vi "BATTERY EMULATOR.vi"() -> ()   [LabVIEW 2018]
uses:
  17a302df-ff61-441d-8d7b-7ff2f5324251.vi
  <vilib>/xnet/xnet.llb/XNET Create Session (Signal Input Single-point).vi
  <vilib>/xnet/xnet.llb/XNET Read (Signal Single-point).vi
panel:
  in  "READ DATA":bool
  out "CP POWER":string
  out "CP CURRENT":string
  out "CP VOLTAGE":string
  out "CI POWER":string
  out "CI CURRENT":string
  out "CI VOLTAGE":string
  out "CV POWER":string
  out "CV CURRENT":string
  out "CV VOLTAGE":string
  out "CONTROL SELECTION":string
  out "HVHC SELECTION":string
  in  "CP POWER":string
  in  "CP CURRENT":string
  in  "CP VOLTAGE":string
  in  "CI POWER":string
  in  "CI CURRENT":string
  in  "CI VOLTAGE":string
  in  "CV POWER":string
  in  "CV CURRENT":string
  in  "CV VOLTAGE":string
  in  "CONTROL SELECTION":string(combo)
  in  "HVHC SELECTION":string(combo)
  out "Headline":string
  in  "Save Button":bool
  in  "MODEL SELECTION":string(combo)
  # "BATTERY EMULATOR CONTROLS"
  # "BATTERY EMULATOR DATA"
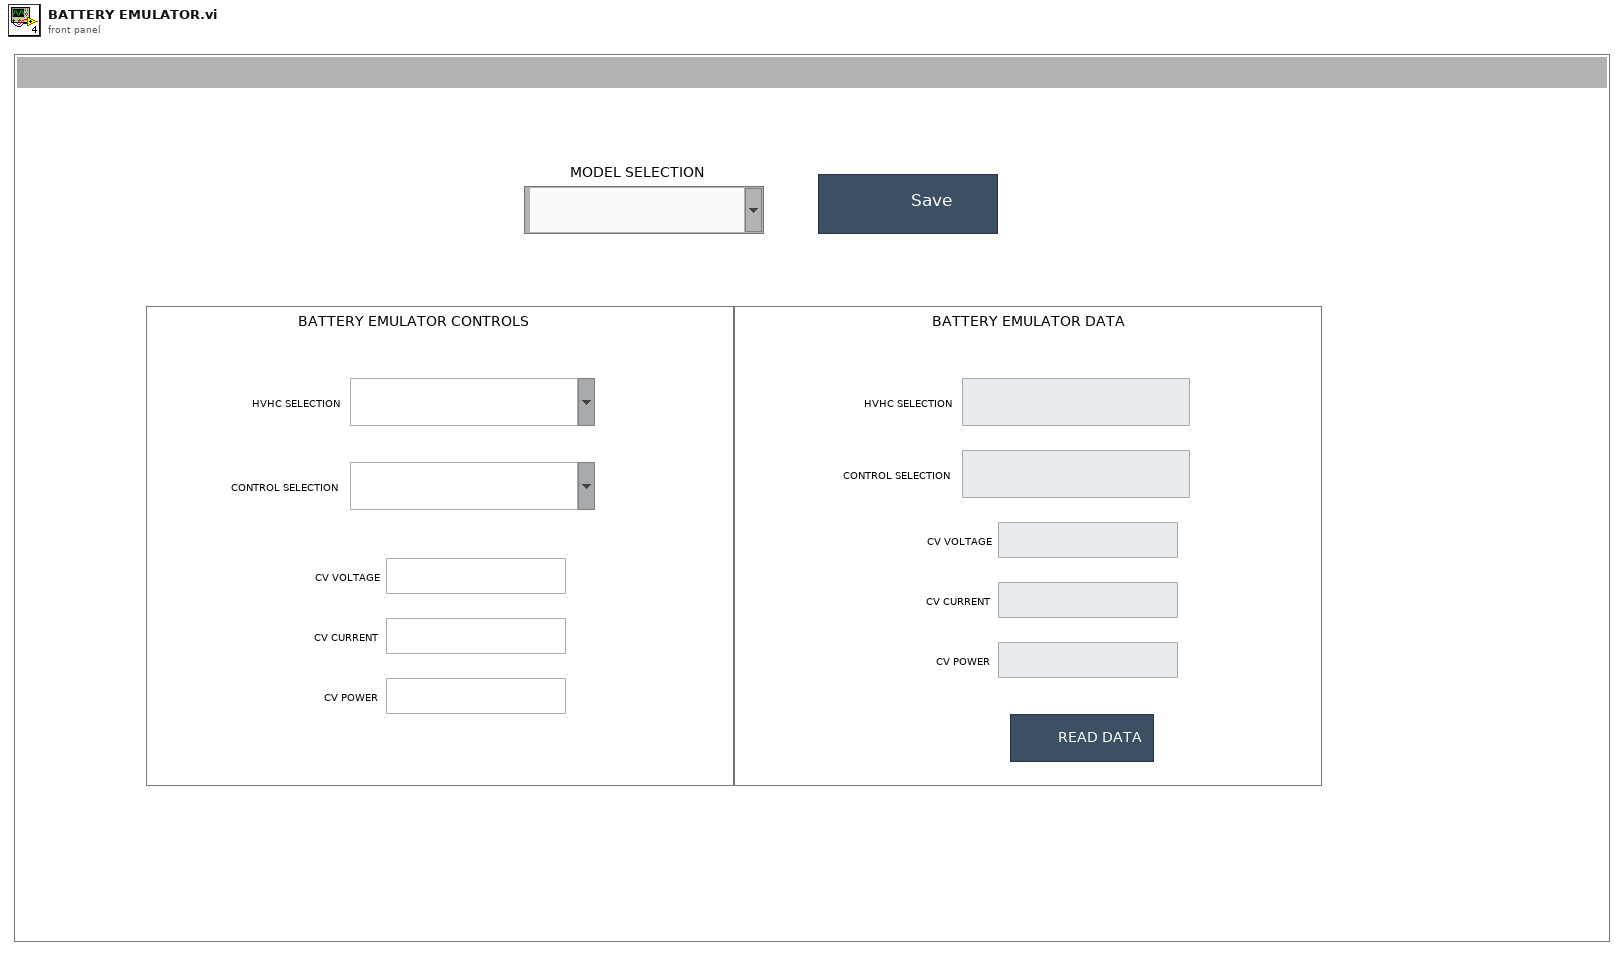
[diagram p1: front panel]
types:
  T1 = enum32{"Invalid", "Standard", "Closed", "Hidden", "Minimized", "Maximized"}
  T2 = enum32{"invalid app kind", "Development System", "Run Time System", "Student Edition", "Embedded LabVIEW", "Evaluation", "Custom"}
  T3 = cluster{"Core":cluster{"Current VI Reference":refnum<vi>, "Close Panel on Exit?":bool}, "Your Boolean data":bool, "Your string data":string, "BATTERY EMULATOR":cluster{"HVHC SELECT":string, "CONTROL SELECTION":string, "CV VOLTAGE":string, "CV CURRENT":string, "CV POWER":string, "CI VOLTAGE":string, "CI CURRENT":string, "CI POWER":string, "CP VOLTAGE":string, "CP CURRENT":string, "CP POWER":string}, "File paths":cluster{"Base file path":path, "Model File path":path}}
  T4 = cluster{"HVHC SELECT":string, "CONTROL SELECTION":string, "CV VOLTAGE":string, "CV CURRENT":string, "CV POWER":string, "CI VOLTAGE":string, "CI CURRENT":string, "CI POWER":string, "CP VOLTAGE":string, "CP CURRENT":string, "CP POWER":string}
  T5 = cluster{"Base file path":path, "Model File path":path}
  T6 = cluster{"Current VI Reference":refnum<vi>, "Close Panel on Exit?":bool}
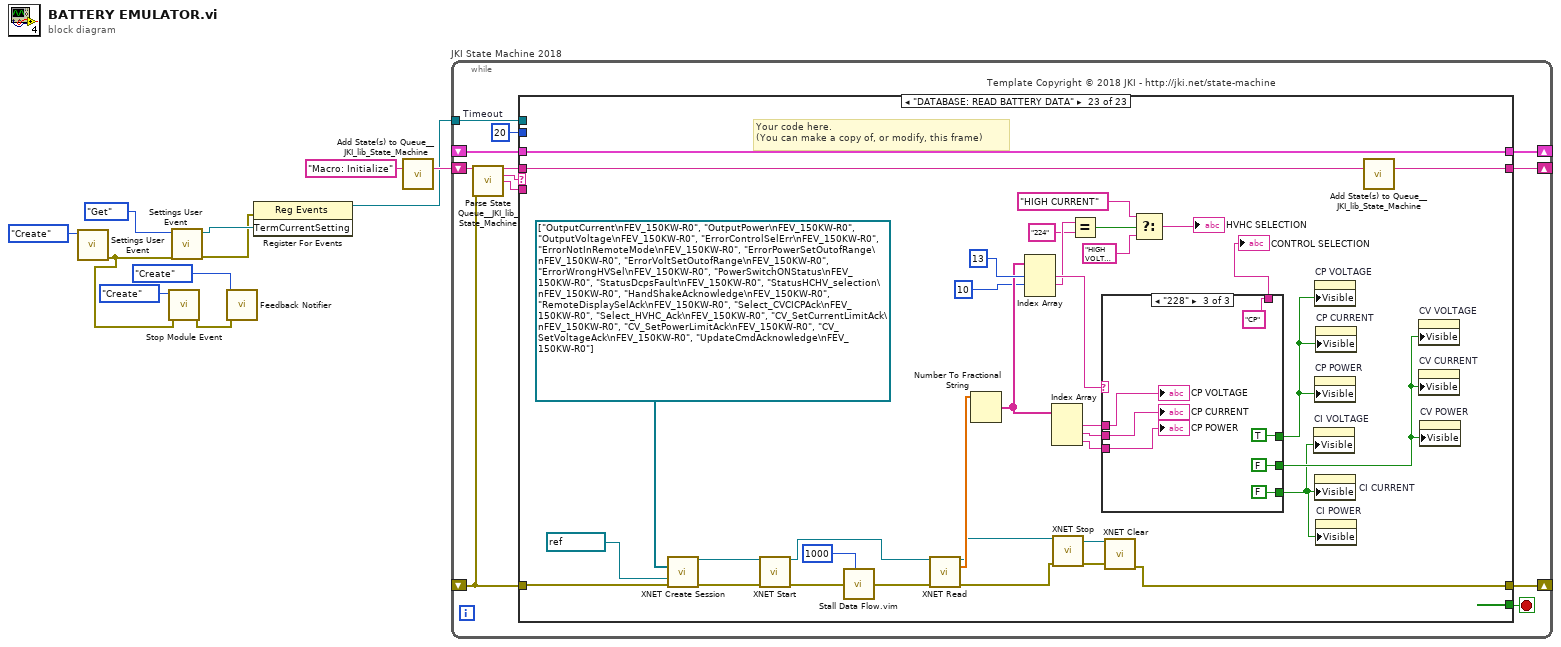
[diagram p0: block diagram]
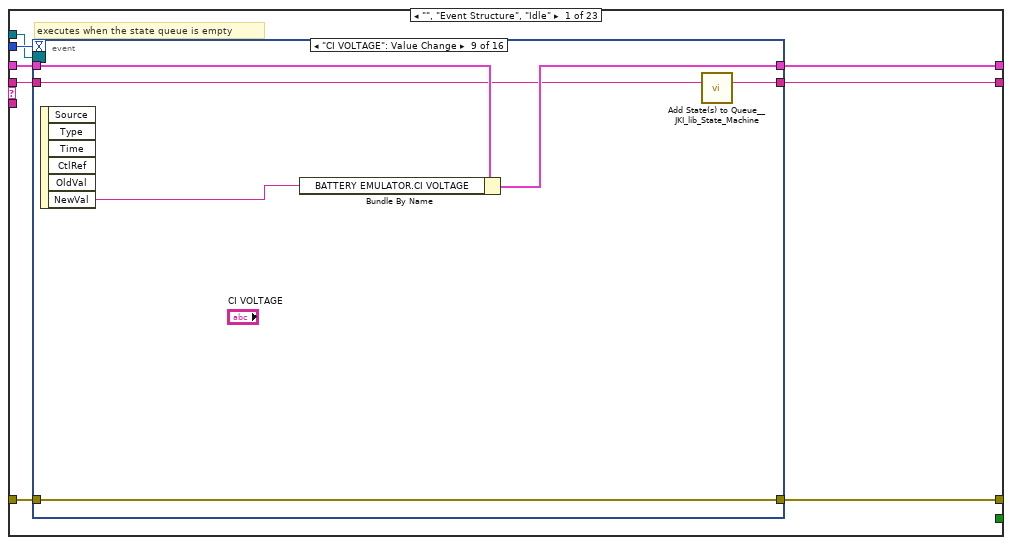
[diagram p2: hidden frame]
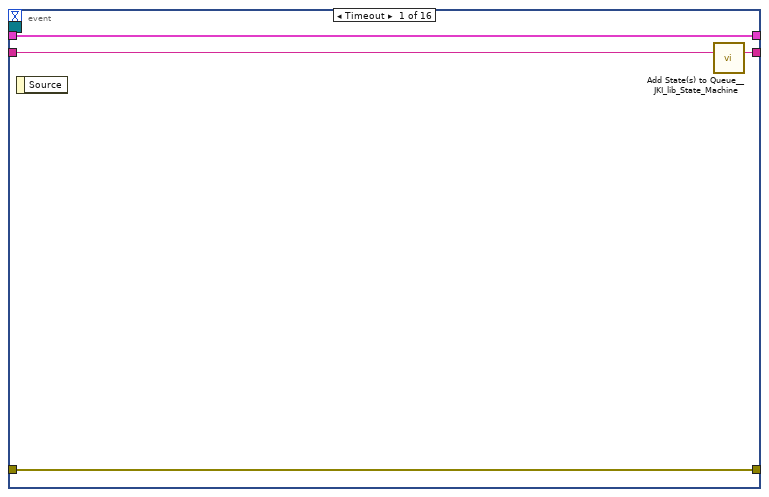
[diagram p3: hidden frame]
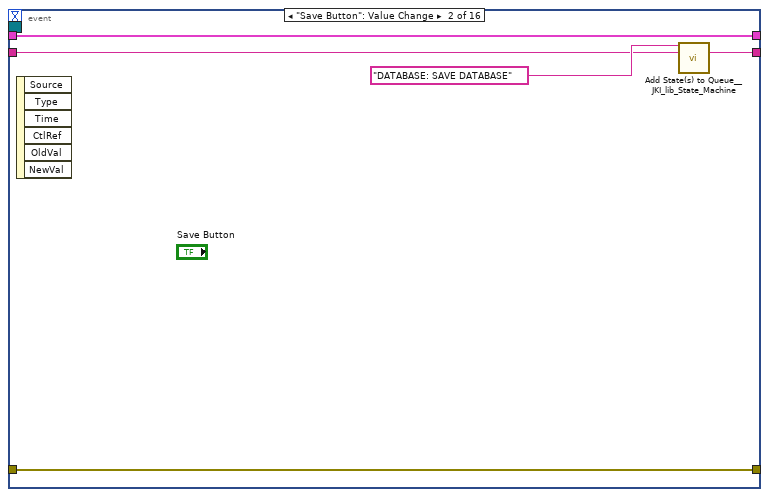
[diagram p4: hidden frame]
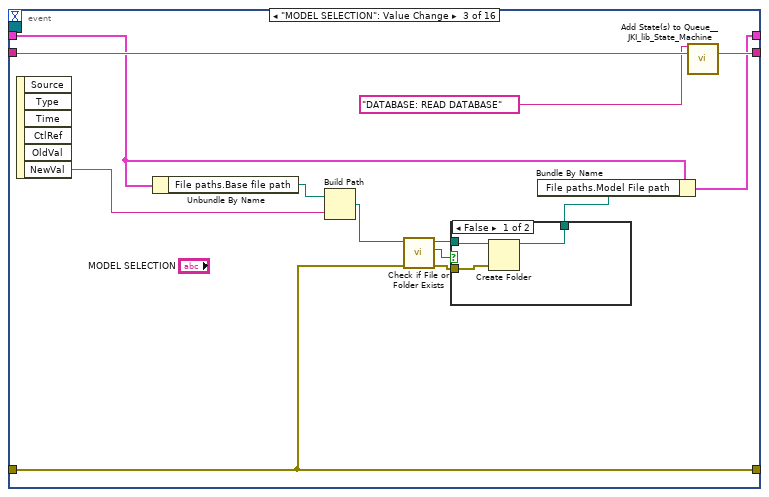
[diagram p5: hidden frame]
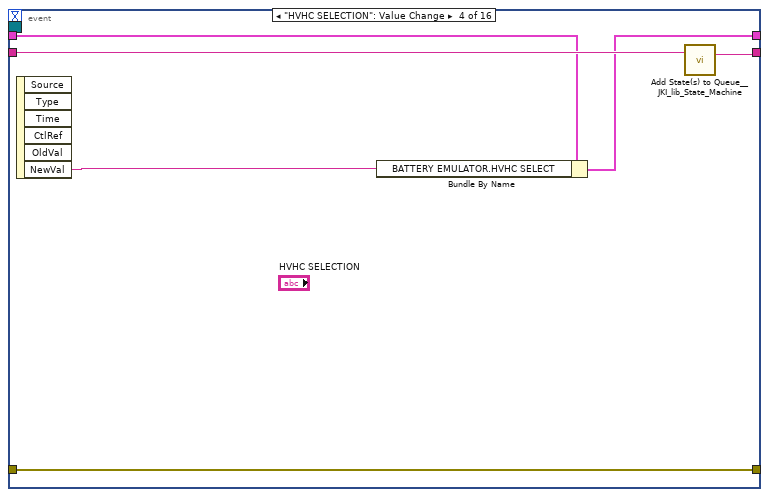
[diagram p7: hidden frame]
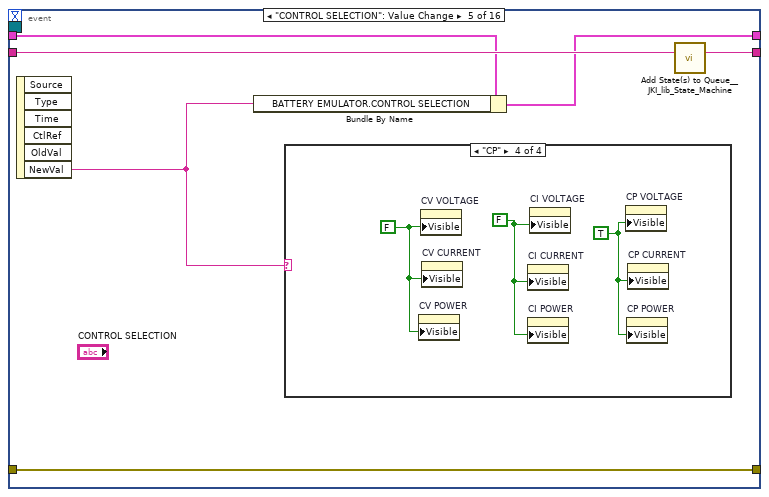
[diagram p8: hidden frame]
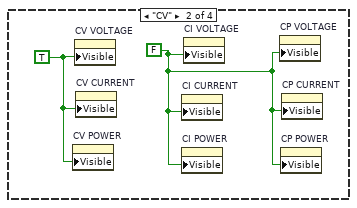
[diagram p10: hidden frame]
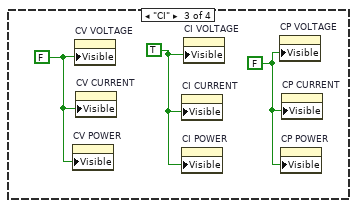
[diagram p11: hidden frame]
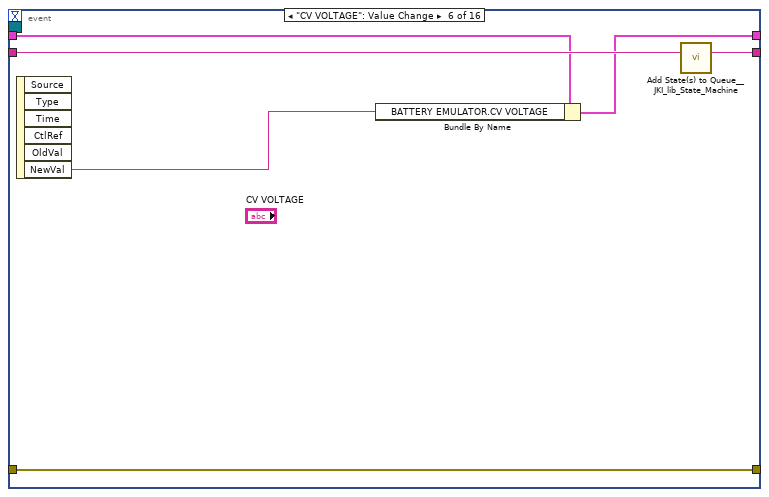
[diagram p12: hidden frame]
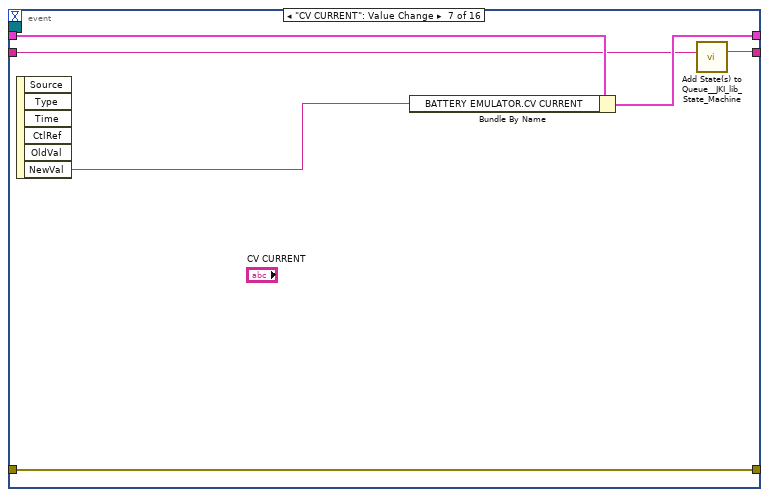
[diagram p13: hidden frame]
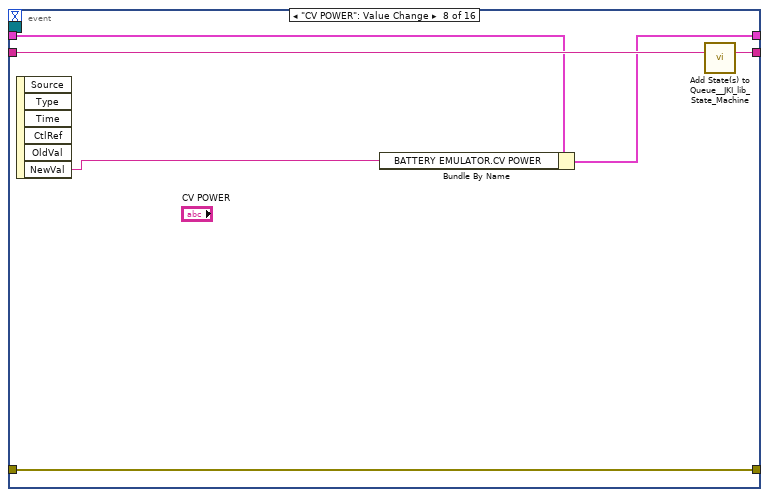
[diagram p14: hidden frame]
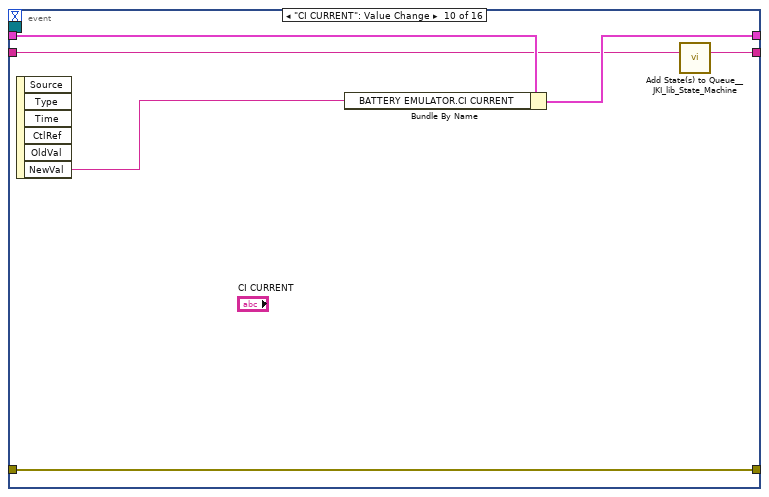
[diagram p15: hidden frame]
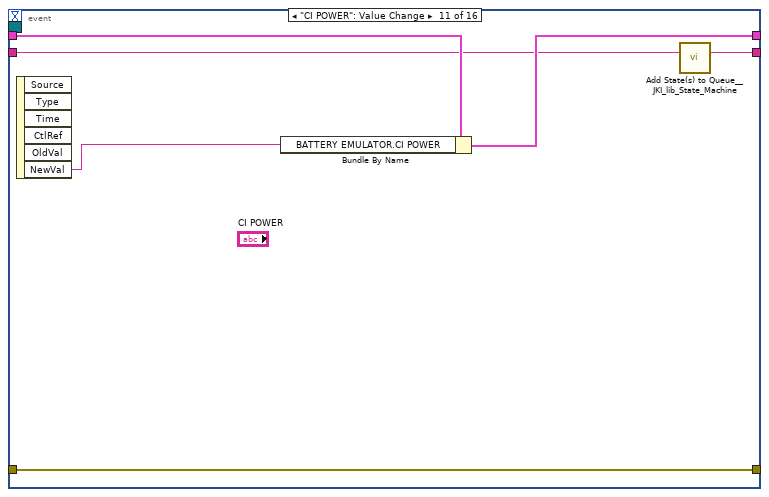
[diagram p16: hidden frame]
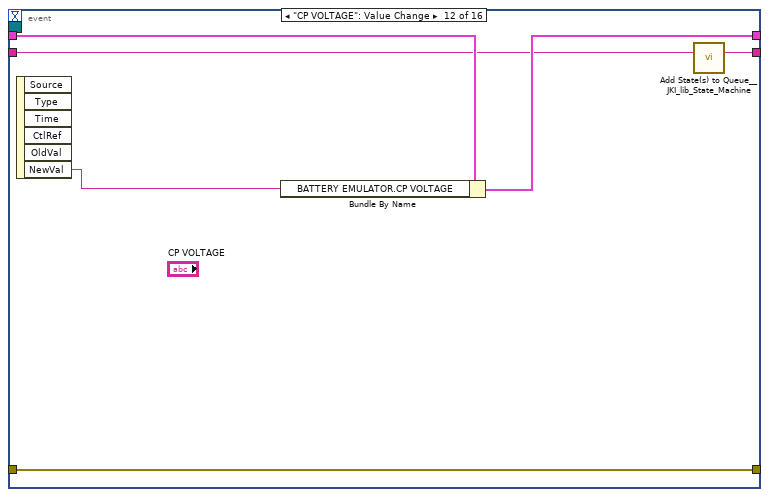
[diagram p17: hidden frame]
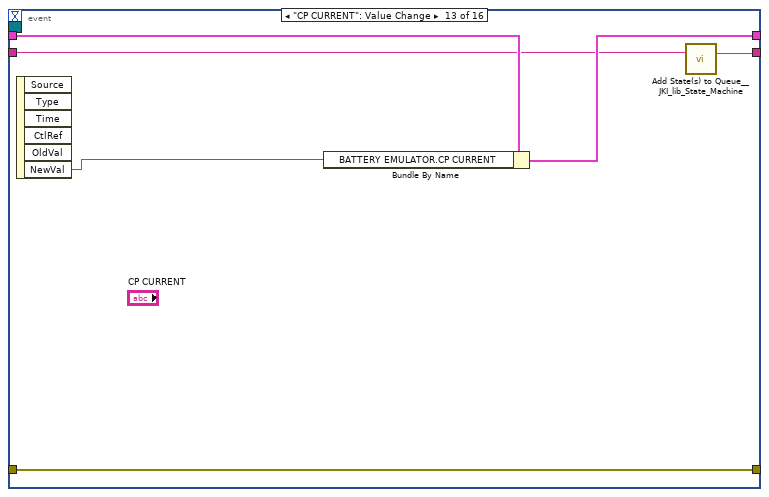
[diagram p18: hidden frame]
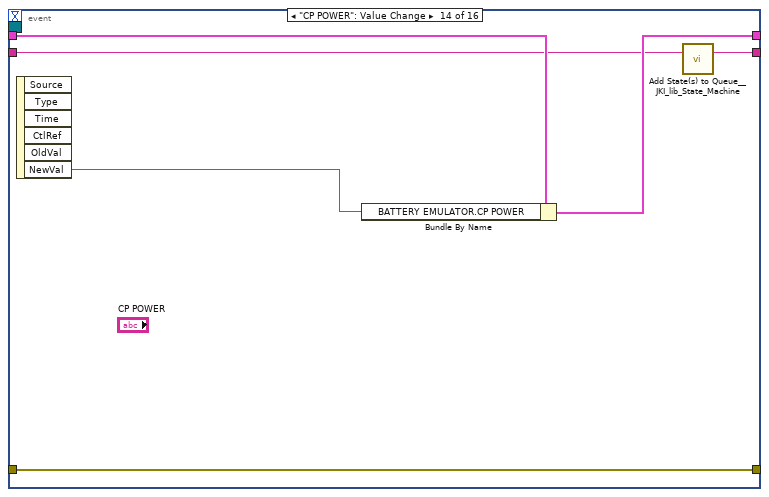
[diagram p19: hidden frame]
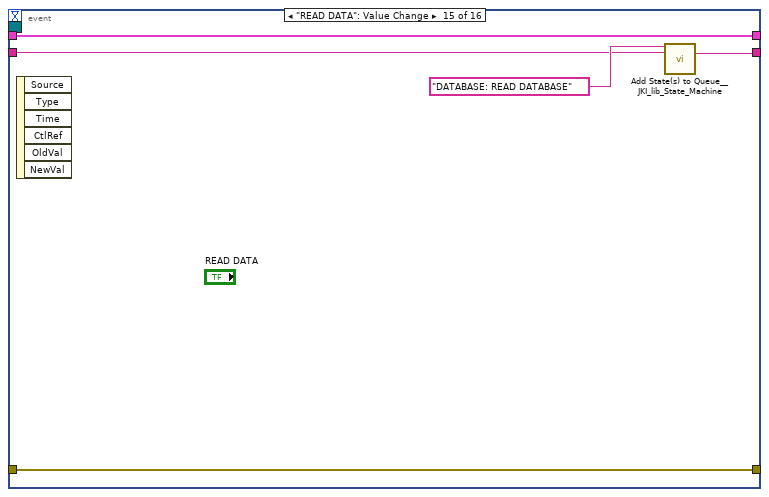
[diagram p20: hidden frame]
diagram:
  n1 = call "Settings User Event.vi"("Action"=enum16{"Create", "Get", "Destroy"}."Create") -> ("error out"=w4:errorcluster)  [unwired: 9 in, 1 out]
  n2 = call "Stop Module Event.vi"("error in (no error)"=w4, "Action"=enum16{"Create", "Get", "Destroy"}."Create") -> ("error out"=w3:errorcluster)  [unwired: 8 in, 1 out]
  n3 = call "Settings User Event.vi"("error in (no error)"=w4, "Action"=enum16{"Create", "Get", "Destroy"}."Get") -> ("error out"=w6:errorcluster, "TermCurrentSetting"=w7:refnum<user-event>)  [unwired: 8 in]
  n4 = call "Feedback Notifier.vi"("error in (no error)"=w3, "Action"=enum16{"Create", "Get", "Destroy"}."Create") -> ()  [unwired: 8 in, 2 out]
  n5 = register-events(error in=w6, w7) -> (reference out=w1:refnum<event-registration>)  [unwired: 1 in, 1 out]
  n6 = call <vilib>:"Add State(s) to Queue__JKI_lib_State_Machine.vi"("State(s) in (\"\")"="Macro: Initialize") -> ("States Out"=w11:string)  [unwired: 14 in]
  n7 = while "JKI State Machine 2018" {
    shift-right: [w16] -> _
    shift-left: _ -> [w15]
    shift-right: [w19] -> _
    shift-left: _ -> [w13]
    shift-right: [w18] -> _
    shift-left: w11 -> [w20]
    tunnel: w1 -> [w12]
    stop <- w17 stop-if-true
    w14 = 20  # Timeout
    # "Template Copyright © 2018 JKI - http://jki.net/state-machine"
    n8 = call <vilib>:"Parse State Queue__JKI_lib_State_Machine.vi"("State Queue"=w20, "Error In (no error)"=w13) -> ("Remaining States"=w22:string, "Current State"=w23:string, "Arguments"=w21:string)  [unwired: 11 in]
    n9 = case shown="\"DATABASE: READ BATTERY DATA\"" w23 {
      selector: w23 -> [_ _ w147 _ _ _ _ _ _ _ _ _ _ _ _ _ _ _ _ _ _ _ _]
      tunnel: w22 -> [w31 w146 w151 w170 w176 w181 w185 w194 w200 w204 w208 w214 w218 w233 w239 w250 w319 w324 w334 w338 w348 w373 w408]
      tunnel: w21 -> [_ _ _ _ _ _ _ _ _ _ _ _ _ _ w234 w244 _ _ _ _ _ _ _]
      tunnel: w15 -> [w29 w143 w149 w163 w173 w179 w182 _ w195 w201 w206 w212 w215 w227 w237 w246 w316 w321 w331 w335 w346 w371 w406]
      tunnel: [w28 w144 w153 w167 errorcluster {"status"=FALSE, "code"=0, "source"=""} ("error out") w178 w183 w191 w196 w202 w205 w209 w216 w228 w235 w247 w317 w322 w332 w336 w341 w366 w374] -> w19
      tunnel: w13 -> [w27 w144 w152 w167 w172 w178 w183 w191 w197 w202 w205 w210 w216 w225 w236 w248 w317 w322 w332 w336 w345 w370 w397]
      tunnel: [w30 w145 w150 w169 w175 w180 w184 w193 w199 w203 w207 w213 w217 w232 w238 w249 w318 w323 w333 w337 w347 w372 w407] -> w18
      tunnel: [_ _ _ _ _ TRUE _ _ _ _ _ _ _ _ _ _ _ _ _ _ _ _ _] -> w17
      tunnel: [w26 w143 w149 w168 w173 w179 w182 w192 w195 w201 w206 w212 w215 w226 w237 w246 w316 w321 w331 w335 w346 w371 w406] -> w16
      tunnel: w14 -> [w25 _ _ _ _ _ _ _ _ _ _ _ _ _ _ _ _ _ _ _ _ _ _]
      tunnel: w12 -> [w24 _ _ _ _ _ _ _ _ _ _ w211 _ _ _ _ _ _ _ _ _ _ _]
      frame "", "Event Structure", "Idle" {
        # "executes when the state queue is empty"
        n10 = event shown="[8] \"CI VOLTAGE\": Value Change" {
          selector: w24 -> [_ _ _ _ _ _ _ _ _ _ _ _ _ _ _ _]
          dyn-events: _ -> [_ _ _ _ _ _ _ _ _ _ _ _ _ _ _ _]
          timeout: w25 -> [_ _ _ _ _ _ _ _ _ _ _ _ _ _ _ _]
          tunnel: w31 -> [w35 w37 w52 w62 w67 w82 w85 w93 w97 w103 w108 w114 w120 w126 w134 w142]
          tunnel: [w34 w38 w53 w63 w68 w83 w86 w94 w98 w104 w109 w115 w121 w127 w135 w141] -> w30
          tunnel: w29 -> [w32 w39 w48 w61 w66 w81 w89 w92 w101 w106 w112 w118 w124 w130 w133 w139]
          tunnel: [w33 w36 w45 w58 w69 w78 w84 w95 w96 w107 w113 w119 w125 w131 w132 w140] -> w28
          tunnel: w27 -> [w33 w36 w45 w58 w69 w78 w84 w95 w96 w107 w113 w119 w125 w131 w132 w140]
          tunnel: [w32 w39 w47 w59 w65 w79 w88 w91 w100 w105 w110 w117 w123 w129 w133 w139] -> w26
          event Timeout {
            n11 = event-data() -> ()  [unwired: 1 in, 1 out]
            n12 = call <vilib>:"Add State(s) to Queue__JKI_lib_State_Machine.vi"("State(s) in (\"\")"=w35) -> ("States Out"=w34:string)  [unwired: 14 in]
          }
          event "Save Button": Value Change {
            n13 = event-data() -> ()  [unwired: 1 in, 6 out]
            n14 = call <vilib>:"Add State(s) to Queue__JKI_lib_State_Machine.vi"("State(s) in Front (\"\")"="DATABASE: SAVE DATABASE", "State(s) in (\"\")"=w37) -> ("States Out"=w38:string)  [unwired: 13 in]
          }
          event "MODEL SELECTION": Value Change {
            n15 = event-data() -> ("NewVal"=w49:string)  [unwired: 1 in, 5 out]
            n16 = Unbundle By Name(w48) -> ("File paths.Base file path"=w50:path)
            n17 = Build Path(base path=w50, name or relative path=w49) -> (appended path=w46:path)
            n18 = call <vilib>:"Check if File or Folder Exists.vi"("error in (no error)"=w45, "path"=w46) -> ("error out"=w43:errorcluster, "file or folder exists?"=w42:bool, "dup path"=w44:path)  [unwired: 7 in]
            n19 = case shown="False" w42 {
              tunnel: w44 -> [w55 w57]
              tunnel: w43 -> [w56 _]
              tunnel: [w54 w57] -> w41
              frame False {
                n20 = Create Folder(path (use dialog)=w55, error in=w56) -> (created path=w54:path)  [unwired: 1 in, 2 out]
              }
              frame True {
              }
            }
            n21 = Bundle By Name(cluster=w48, "File paths.Model File path"=w41) -> (w47:T3)
            n22 = call <vilib>:"Add State(s) to Queue__JKI_lib_State_Machine.vi"("State(s) in Front (\"\")"="DATABASE: READ DATABASE", "State(s) in (\"\")"=w52) -> ("States Out"=w53:string)  [unwired: 13 in]
          }
          event "HVHC SELECTION": Value Change {
            n23 = event-data() -> ("NewVal"=w60:string)  [unwired: 1 in, 5 out]
            n24 = Bundle By Name(cluster=w61, "BATTERY EMULATOR.HVHC SELECT"=w60) -> (w59:T3)
            n25 = call <vilib>:"Add State(s) to Queue__JKI_lib_State_Machine.vi"("State(s) in (\"\")"=w62) -> ("States Out"=w63:string)  [unwired: 14 in]
          }
          event "CONTROL SELECTION": Value Change {
            n26 = event-data() -> ("NewVal"=w64:string)  [unwired: 1 in, 5 out]
            n27 = Bundle By Name(cluster=w66, "BATTERY EMULATOR.CONTROL SELECTION"=w64) -> (w65:T3)
            n28 = case shown="\"CP\"" w64 {
              frame "False", Default {
              }
              frame "CV" {
                w70 = FALSE ("Visible")
                w71 = TRUE ("Visible")
                n29 = property on="CV POWER" class="Str"("Visible"=w71) -> ()  [unwired: 2 in, 2 out]
                n30 = property on="CV VOLTAGE" class="Str"("Visible"=w71) -> ()  [unwired: 2 in, 2 out]
                n31 = property on="CV CURRENT" class="Str"("Visible"=w71) -> ()  [unwired: 2 in, 2 out]
                n32 = property on="CI CURRENT" class="Str"("Visible"=w70) -> ()  [unwired: 2 in, 2 out]
                n33 = property on="CI POWER" class="Str"("Visible"=w70) -> ()  [unwired: 2 in, 2 out]
                n34 = property on="CI VOLTAGE" class="Str"("Visible"=w70) -> ()  [unwired: 2 in, 2 out]
                n35 = property on="CP VOLTAGE" class="Str"("Visible"=w70) -> ()  [unwired: 2 in, 2 out]
                n36 = property on="CP POWER" class="Str"("Visible"=w70) -> ()  [unwired: 2 in, 2 out]
                n37 = property on="CP CURRENT" class="Str"("Visible"=w70) -> ()  [unwired: 2 in, 2 out]
              }
              frame "CI" {
                w72 = FALSE ("Visible")
                w73 = TRUE ("Visible")
                w74 = FALSE ("Visible")
                n38 = property on="CV POWER" class="Str"("Visible"=w74) -> ()  [unwired: 2 in, 2 out]
                n39 = property on="CV VOLTAGE" class="Str"("Visible"=w74) -> ()  [unwired: 2 in, 2 out]
                n40 = property on="CV CURRENT" class="Str"("Visible"=w74) -> ()  [unwired: 2 in, 2 out]
                n41 = property on="CI CURRENT" class="Str"("Visible"=w73) -> ()  [unwired: 2 in, 2 out]
                n42 = property on="CI POWER" class="Str"("Visible"=w73) -> ()  [unwired: 2 in, 2 out]
                n43 = property on="CI VOLTAGE" class="Str"("Visible"=w73) -> ()  [unwired: 2 in, 2 out]
                n44 = property on="CP VOLTAGE" class="Str"("Visible"=w72) -> ()  [unwired: 2 in, 2 out]
                n45 = property on="CP POWER" class="Str"("Visible"=w72) -> ()  [unwired: 2 in, 2 out]
                n46 = property on="CP CURRENT" class="Str"("Visible"=w72) -> ()  [unwired: 2 in, 2 out]
              }
              frame "CP" {
                w75 = TRUE ("Visible")
                w76 = FALSE ("Visible")
                w77 = FALSE ("Visible")
                n47 = property on="CV POWER" class="Str"("Visible"=w77) -> ()  [unwired: 2 in, 2 out]
                n48 = property on="CV VOLTAGE" class="Str"("Visible"=w77) -> ()  [unwired: 2 in, 2 out]
                n49 = property on="CV CURRENT" class="Str"("Visible"=w77) -> ()  [unwired: 2 in, 2 out]
                n50 = property on="CI CURRENT" class="Str"("Visible"=w76) -> ()  [unwired: 2 in, 2 out]
                n51 = property on="CI POWER" class="Str"("Visible"=w76) -> ()  [unwired: 2 in, 2 out]
                n52 = property on="CI VOLTAGE" class="Str"("Visible"=w76) -> ()  [unwired: 2 in, 2 out]
                n53 = property on="CP VOLTAGE" class="Str"("Visible"=w75) -> ()  [unwired: 2 in, 2 out]
                n54 = property on="CP POWER" class="Str"("Visible"=w75) -> ()  [unwired: 2 in, 2 out]
                n55 = property on="CP CURRENT" class="Str"("Visible"=w75) -> ()  [unwired: 2 in, 2 out]
              }
            }
            n56 = call <vilib>:"Add State(s) to Queue__JKI_lib_State_Machine.vi"("State(s) in (\"\")"=w67) -> ("States Out"=w68:string)  [unwired: 14 in]
          }
          event "CV VOLTAGE": Value Change {
            n57 = event-data() -> ("NewVal"=w80:string)  [unwired: 1 in, 5 out]
            n58 = Bundle By Name(cluster=w81, "BATTERY EMULATOR.CV VOLTAGE"=w80) -> (w79:T3)
            n59 = call <vilib>:"Add State(s) to Queue__JKI_lib_State_Machine.vi"("State(s) in (\"\")"=w82) -> ("States Out"=w83:string)  [unwired: 14 in]
          }
          event "CV CURRENT": Value Change {
            n60 = event-data() -> ("NewVal"=w87:string)  [unwired: 1 in, 5 out]
            n61 = Bundle By Name(cluster=w89, "BATTERY EMULATOR.CV CURRENT"=w87) -> (w88:T3)
            n62 = call <vilib>:"Add State(s) to Queue__JKI_lib_State_Machine.vi"("State(s) in (\"\")"=w85) -> ("States Out"=w86:string)  [unwired: 14 in]
          }
          event "CV POWER": Value Change {
            n63 = event-data() -> ("NewVal"=w90:string)  [unwired: 1 in, 5 out]
            n64 = Bundle By Name(cluster=w92, "BATTERY EMULATOR.CV POWER"=w90) -> (w91:T3)
            n65 = call <vilib>:"Add State(s) to Queue__JKI_lib_State_Machine.vi"("State(s) in (\"\")"=w93) -> ("States Out"=w94:string)  [unwired: 14 in]
          }
          event "CI VOLTAGE": Value Change {
            n66 = event-data() -> ("NewVal"=w99:string)  [unwired: 1 in, 5 out]
            n67 = Bundle By Name(cluster=w101, "BATTERY EMULATOR.CI VOLTAGE"=w99) -> (w100:T3)
            n68 = call <vilib>:"Add State(s) to Queue__JKI_lib_State_Machine.vi"("State(s) in (\"\")"=w97) -> ("States Out"=w98:string)  [unwired: 14 in]
          }
          event "CI CURRENT": Value Change {
            n69 = event-data() -> ("NewVal"=w102:string)  [unwired: 1 in, 5 out]
            n70 = Bundle By Name(cluster=w106, "BATTERY EMULATOR.CI CURRENT"=w102) -> (w105:T3)
            n71 = call <vilib>:"Add State(s) to Queue__JKI_lib_State_Machine.vi"("State(s) in (\"\")"=w103) -> ("States Out"=w104:string)  [unwired: 14 in]
          }
          event "CI POWER": Value Change {
            n72 = event-data() -> ("NewVal"=w111:string)  [unwired: 1 in, 5 out]
            n73 = Bundle By Name(cluster=w112, "BATTERY EMULATOR.CI POWER"=w111) -> (w110:T3)
            n74 = call <vilib>:"Add State(s) to Queue__JKI_lib_State_Machine.vi"("State(s) in (\"\")"=w108) -> ("States Out"=w109:string)  [unwired: 14 in]
          }
          event "CP VOLTAGE": Value Change {
            n75 = event-data() -> ("NewVal"=w116:string)  [unwired: 1 in, 5 out]
            n76 = Bundle By Name(cluster=w118, "BATTERY EMULATOR.CP VOLTAGE"=w116) -> (w117:T3)
            n77 = call <vilib>:"Add State(s) to Queue__JKI_lib_State_Machine.vi"("State(s) in (\"\")"=w114) -> ("States Out"=w115:string)  [unwired: 14 in]
          }
          event "CP CURRENT": Value Change {
            n78 = event-data() -> ("NewVal"=w122:string)  [unwired: 1 in, 5 out]
            n79 = Bundle By Name(cluster=w124, "BATTERY EMULATOR.CP CURRENT"=w122) -> (w123:T3)
            n80 = call <vilib>:"Add State(s) to Queue__JKI_lib_State_Machine.vi"("State(s) in (\"\")"=w120) -> ("States Out"=w121:string)  [unwired: 14 in]
          }
          event "CP POWER": Value Change {
            n81 = event-data() -> ("NewVal"=w128:string)  [unwired: 1 in, 5 out]
            n82 = Bundle By Name(cluster=w130, "BATTERY EMULATOR.CP POWER"=w128) -> (w129:T3)
            n83 = call <vilib>:"Add State(s) to Queue__JKI_lib_State_Machine.vi"("State(s) in (\"\")"=w126) -> ("States Out"=w127:string)  [unwired: 14 in]
          }
          event "READ DATA": Value Change {
            n84 = event-data() -> ()  [unwired: 1 in, 6 out]
            n85 = call <vilib>:"Add State(s) to Queue__JKI_lib_State_Machine.vi"("State(s) in Front (\"\")"="DATABASE: READ DATABASE", "State(s) in (\"\")"=w134) -> ("States Out"=w135:string)  [unwired: 13 in]
          }
          event Panel Close? {
            # "Discard the event because we'll close the front panel ourselves in Macro: Exit"
            # "Close Panel button (pressed) Event\n(this executes Macro: Exit to terminate the VI)"
            n86 = event-data() -> ()  [unwired: 1 in, 1 out]
            n87 = event-data("Discard?"=TRUE) -> ()  [unwired: 1 in, 1 out]
            n88 = call <vilib>:"Add State(s) to Queue__JKI_lib_State_Machine.vi"("State(s) in Front (\"\")"="Macro: Exit", "State(s) in (\"\")"=w142) -> ("States Out"=w141:string)  [unwired: 13 in]
          }
        }
      }
      frame "---------- Core ----------" {
        # "Do not put any code in this frame.\n(it is a separator no-op)"
        n89 = call <vilib>:"Add State(s) to Queue__JKI_lib_State_Machine.vi"("State(s) in (\"\")"=w146) -> ("States Out"=w145:string)  [unwired: 14 in]
      }
      frame Default {
        w156 = 42 items=["No error", "Argument error", "Memory is full", "Out of zone", "End of file", "File already open", "Generic file I/O error", "File not found", "File permission error", "Disk is full", "Duplicate path", "Too many files open", "System feature not enabled", "Resource file not found", "Cannot add resource", "Resource not found", "Image not found", "Image memory error", "Pen does not exist", "Config type invalid", "Config token not found", "Config parse error", "Config memory error", "Bad external code format", "Bad external code offset", "External code not present", "Null window", "Destroy window error", "Null menu", "Print aborted", "Bad print record", "Print driver error", "Windows error during printing", "Memory error during printing", "Print dialog error", "Generic print error", "Invalid device refnum", "Device not found", "Device parameter error", "Device unit error", "Cannot open device", "Device call aborted", "Generic error", "Cancelled by user", "Object ID too low", "Object ID too high", "Object not in heap", "Unknown heap", "Unknown object (invalid DefProc)", "Unknown object (DefProc not in table)", "Message out of range", "Invalid (null) method", "Unknown message", "Manager call not supported", "Bad address", "Network operation in progress", "Network operation timed out", "Connection is busy", "Network attribute not supported", "Network error", "Address in use", "System out of memory", "Connection aborted", "Connection refused", "Not connected", "Already connected", "Connection closed", "Initialization error (interapplication manager)", "Bad occurrence", "Wait on unbound occurrence handler", "Occurrence queue overflow", "Datalog type conflict", "Unused", "Unrecognized type (interapplication manager)", "Memory corrupt", "Failed to make temporary DLL", "Old CIN version", "Drag socket not found", "Failed to load drop-object", "Failed to register OLE object", "Failed to release OLE object", "Format specifier type mismatch", "Unknown format specifier", "Too few format specifiers", "Too many format specifiers", "Scan failed", "Newer CIN version", "Error converting to variant", "Runtime menu error", "Password tampered", "Variant attribute not found", "Incompatible variant data type", "Event data is not available", "Event Store is not present", "Occurrence is not found", "Event Queue is not created", "Event info is not available", "Refnum passed is NULL", "Error retrieving Class GUID", "Error retrieving CoClass GUID", "Error retrieving TypeLib GUID.", "Bad built application magic bytes.", "Specific driver is different from the specific driver associated with the Logical Name.", "There is no session opened to the class driver.", "Max Error", "MAX - Error with config objects", "MAX - Error loading configuration", "MAX - Group not supported"]
        # "Current State"
        # "Do not delete, rename, or modify this frame.\n(this is used to capture unhandled states and typos)"
        # "Handle mistyped state name (developer tool)"
        n90 = Format Into String(format string="Software Exception: Unhandled State \"%s\"." ("message"), error in=w152, w147) -> (resulting string=w155:string, error out=w154:errorcluster)  [unwired: 1 in]
        n91 = call <vilib>:"Error Cluster From Error Code.vi"("show call chain? (False)"=TRUE, "error in (no error)"=w154, "error message (\"\")"=w155, "error code (0)"=w156) -> ("error out"=w153:errorcluster)  [unwired: 5 in]
        n92 = call <vilib>:"Add State(s) to Queue__JKI_lib_State_Machine.vi"("State(s) in (\"\")"=w151) -> ("States Out"=w150:string)  [unwired: 14 in]
      }
      frame "Initialize Core Data" {
        # "Do not delete, rename, or modify this frame.\n(this is used to determine panel behavior on exit)"
        # "originally closed?"
        # "exe?"
        # "If panel starts closed or is an EXE, then close it when we exit"
        n93 = property class="VI"() -> ("FP.State"=w160:T1)  [unwired: 2 in, 2 out]
        n94 = property class="App"() -> ("App.Kind"=w166:T2)  [unwired: 2 in, 2 out]
        n95 = control-ref of="Current VI Reference"() -> (w161:refnum<vi>)
        n96 = Equal?(x=w160, y=T1."Closed" ("Front Panel Window:State")) -> (x = y?=w158:bool)
        n97 = Equal?(x=w166, y=T2."Run Time System" ("Application:Kind")) -> (x = y?=w164:bool)
        n98 = Or(x=w158, y=w164) -> (x .or. y?=w162:bool)
        n99 = Bundle By Name(cluster=w163, "Core.Current VI Reference"=w161, "Core.Close Panel on Exit?"=w162) -> (w168:T3)
        n100 = call <vilib>:"Add State(s) to Queue__JKI_lib_State_Machine.vi"("State(s) in (\"\")"=w170) -> ("States Out"=w169:string)  [unwired: 14 in]
      }
      frame "Error Handler" {
        # "Unhandled Error -- Display it"
        # "Handle any errors here.\nYou can also output any states to clean-up after errors occur"
        # "Clear error"
        n101 = call <vilib>:"General Error Handler.vi"("error in (no error)"=w172) -> ()  [unwired: 10 in, 5 out]
        n102 = call <vilib>:"Add State(s) to Queue__JKI_lib_State_Machine.vi"("State(s) in Front (\"\")"="/* Post Error States", "State(s) in (\"\")"=w176) -> ("States Out"=w175:string)  [unwired: 13 in]
      }
      frame "Exit" {
        # "Do not put any code in this frame.\n(No errors that occur here will be handled.)"
        n103 = call <vilib>:"Add State(s) to Queue__JKI_lib_State_Machine.vi"("State(s) in (\"\")"=w181) -> ("States Out"=w180:string)  [unwired: 14 in]
      }
      frame "---------- Data ----------" {
        # "Do not put any code in this frame.\n(It is a separator no-op. You can make a copy of this frame to create a new Data frame)"
        n104 = call <vilib>:"Add State(s) to Queue__JKI_lib_State_Machine.vi"("State(s) in (\"\")"=w185) -> ("States Out"=w184:string)  [unwired: 14 in]
      }
      frame "Data: Initialize" {
        w186 = T4 {"HVHC SELECT"="", "CONTROL SELECTION"="", "CV VOLTAGE"="", "CV CURRENT"="", "CV POWER"="", "CI VOLTAGE"="", "CI CURRENT"="", "CI POWER"="", "CP VOLTAGE"="", "CP CURRENT"="", "CP POWER"=""}  # BATTERY EMULATOR
        w187 = T5 {"Base file path"=path "", "Model File path"=path ""}  # File paths
        w188 = T6 {"Current VI Reference"=refnum, "Close Panel on Exit?"=FALSE}  # Core
        w190 = TRUE  # Your Boolean data
        w189 = ""  # Your string data
        # "do not delete - used by framework"
        # "Data names and types of shift register data are defined by this bundle."
        # "Initialize the shift-register data, here.\n(data names are defined by what you wire into the bundle function)"
        n105 = Bundle("Core"=w188, "Your Boolean data"=w190, "Your string data"=w189, "BATTERY EMULATOR"=w186, "File paths"=w187) -> (w192:T3)  [unwired: 1 in]
        n106 = call <vilib>:"Add State(s) to Queue__JKI_lib_State_Machine.vi"("State(s) in (\"\")"=w194) -> ("States Out"=w193:string)  [unwired: 14 in]
      }
      frame "Data: Cleanup" {
        # "Cleanup any data and references, here.\n(this is called automatically, by the Macro: Exit)"
        n107 = Unbundle By Name(w195) -> ("Core.Current VI Reference"=w198:refnum<vi>)
        n108 = Close Reference(reference=w198, error in (no error)=w197) -> (error out=w196:errorcluster)
        n109 = call <vilib>:"Add State(s) to Queue__JKI_lib_State_Machine.vi"("State(s) in (\"\")"=w200) -> ("States Out"=w199:string)  [unwired: 14 in]
      }
      frame "---------- Events ----------" {
        # "Do not put any code in this frame.\n(It is a separator no-op. You can make a copy of this frame to create a new UI frame)"
        n110 = call <vilib>:"Add State(s) to Queue__JKI_lib_State_Machine.vi"("State(s) in (\"\")"=w204) -> ("States Out"=w203:string)  [unwired: 14 in]
      }
      frame "Events: Register" {
        # "Do not put any code in this frame.\n(It is a separator no-op. You can make a copy of this frame to create a new UI frame)"
        n111 = call <vilib>:"Add State(s) to Queue__JKI_lib_State_Machine.vi"("State(s) in (\"\")"=w208) -> ("States Out"=w207:string)  [unwired: 14 in]
      }
      frame "Events: Unregister" {
        # "Do not put any code in this frame.\n(It is a separator no-op. You can make a copy of this frame to create a new UI frame)"
        n112 = Unregister For Events(event registration refnum=w211, error in=w210) -> (error out=w209:errorcluster)
        n113 = call <vilib>:"Add State(s) to Queue__JKI_lib_State_Machine.vi"("State(s) in (\"\")"=w214) -> ("States Out"=w213:string)  [unwired: 14 in]
      }
      frame "---------- UI ----------" {
        # "Do not put any code in this frame.\n(It is a separator no-op. You can make a copy of this frame to create a new UI frame)"
        n114 = call <vilib>:"Add State(s) to Queue__JKI_lib_State_Machine.vi"("State(s) in (\"\")"=w218) -> ("States Out"=w217:string)  [unwired: 14 in]
      }
      frame "UI: Initialize" {
        # "Initialize the User Interface, here.\n(this is called automatically, by the Macro: Init)"
        n115 = invoke class="VI" method="Default Vals.Reinit All"(error in=w225) -> (error out=w224:errorcluster)  [unwired: 2 in, 2 out]
        n116 = Current VI's Path() -> (path=w230:path)
        n117 = call "FEV_Strip & Build Path.vi"("Strip Levels"=2, "error in (no error)"=w224, "Build Path"="Data\\Models", "Path In"=w230) -> ("error out"=w228:errorcluster, "New Path Out"=w222:path)  [unwired: 5 in, 1 out]
        n118 = List Folder(path=w222) -> (folder names=w221:string[])  [unwired: 3 in, 3 out]
        n119 = Bundle By Name(cluster=w227, "File paths.Base file path"=w222) -> (w226:T3)
        n120 = property on="MODEL SELECTION" class="CmbBox"("Strings[]"=w221) -> ()  [unwired: 2 in, 2 out]
        n121 = property on="CONTROL SELECTION" class="CmbBox"("Strings[]"=string[] ["CV", "CI", "CP"]) -> ()  [unwired: 2 in, 2 out]
        n122 = property on="HVHC SELECTION" class="CmbBox"("Strings[]"=string[] ["HIGH CURRENT", "HIGH VOLTAGE"]) -> ()  [unwired: 2 in, 2 out]
        n123 = call <vilib>:"Add State(s) to Queue__JKI_lib_State_Machine.vi"("State(s) in (\"\")"=w233) -> ("States Out"=w232:string)  [unwired: 14 in]
        "Headline" <- "Battery Emulator Configuration" ("Headline")
      }
      frame "UI: Cursor Set" {
        # "Argument"
        # "Set and Unset Cursor Busy.\n(Usage: \"UI: Cursor Set >> Busy|Idle\")"
        n124 = case shown="\"Idle\", Default" w234 {
          tunnel: w236 -> [w241 w243]
          tunnel: [w240 w242] -> w235
          frame "Idle", Default {
            n125 = call <vilib>:"Unset Busy.vi"("error in (no error)"=w241) -> ("error out"=w240:errorcluster)  [unwired: 10 in]
          }
          frame "Busy" {
            n126 = call <vilib>:"Set Busy.vi"("error in (no error)"=w243) -> ("error out"=w242:errorcluster)  [unwired: 9 in, 1 out]
          }
        }
        n127 = call <vilib>:"Add State(s) to Queue__JKI_lib_State_Machine.vi"("State(s) in (\"\")"=w239) -> ("States Out"=w238:string)  [unwired: 14 in]
      }
      frame "UI: Front Panel State" {
        # "Argument"
        # "Set Front Panel Open or Closed\n(Usage: \"UI: Front Panel State >> Open|Close\")"
        n128 = Unbundle By Name(w246) -> ("Core.Current VI Reference"=w245:refnum<vi>)
        n129 = case shown="\"Open\", \"Standard\", Default" w244 {
          tunnel: w248 -> [w256 w271 w282 w295 w308]
          tunnel: [w258 w272 w284 w297 w310] -> w247
          tunnel: w245 -> [w257 w269 w283 w296 w309]
          frame "Open", "Standard", Default {
            w251 = T1."Standard" ("State")
            n130 = property class="VI"(reference=w257, error in=w256) -> (reference out=w254:refnum<vi>, error out=w255:errorcluster, "FP.State"=w253:T1)
            n131 = Not Equal?(x=w253, y=w251) -> (x != y?=w252:bool)
            n132 = case shown="True" w252 {
              tunnel: [w262 w264] -> w258
              tunnel: w255 -> [w261 w264]
              tunnel: w254 -> [w260 _]
              tunnel: w251 -> [w259 _]
              frame True {
                n133 = invoke class="VI" method="FP.Open"(reference=w260, error in=w261, "Activate"=TRUE, "State"=w259) -> (error out=w262:errorcluster)  [unwired: 1 in, 4 out]
              }
              frame False {
              }
            }
          }
          frame "Close", "Closed" {
            n134 = property class="VI"(reference=w269, error in=w271) -> (reference out=w268:refnum<vi>, error out=w270:errorcluster, "FP.State"=w266:T1)
            n135 = Not Equal?(x=w266, y=T1."Closed" ("Front Panel Window:State")) -> (x != y?=w265:bool)
            n136 = case shown="True" w265 {
              tunnel: [w273 w276] -> w272
              tunnel: w270 -> [w273 w275]
              tunnel: w268 -> [_ w274]
              frame False {
              }
              frame True {
                n137 = invoke class="VI" method="FP.Close"(reference=w274, error in=w275) -> (error out=w276:errorcluster)  [unwired: 1 in, 2 out]
              }
            }
          }
          frame "Hidden", "Hide" {
            w277 = T1."Hidden" ("State")
            n138 = property class="VI"(reference=w283, error in=w282) -> (reference out=w280:refnum<vi>, error out=w281:errorcluster, "FP.State"=w279:T1)
            n139 = Not Equal?(x=w279, y=w277) -> (x != y?=w278:bool)
            n140 = case shown="True" w278 {
              tunnel: [w288 w289] -> w284
              tunnel: w281 -> [w287 w289]
              tunnel: w280 -> [w286 _]
              tunnel: w277 -> [w285 _]
              frame True {
                n141 = invoke class="VI" method="FP.Open"(reference=w286, error in=w287, "State"=w285) -> (error out=w288:errorcluster)  [unwired: 2 in, 4 out]
              }
              frame False {
              }
            }
          }
          frame "Minimize", "Minimized" {
            w290 = T1."Minimized" ("State")
            n142 = property class="VI"(reference=w296, error in=w295) -> (reference out=w293:refnum<vi>, error out=w294:errorcluster, "FP.State"=w292:T1)
            n143 = Not Equal?(x=w292, y=w290) -> (x != y?=w291:bool)
            n144 = case shown="True" w291 {
              tunnel: [w301 w302] -> w297
              tunnel: w294 -> [w300 w302]
              tunnel: w293 -> [w299 _]
              tunnel: w290 -> [w298 _]
              frame True {
                n145 = invoke class="VI" method="FP.Open"(reference=w299, error in=w300, "State"=w298) -> (error out=w301:errorcluster)  [unwired: 2 in, 4 out]
              }
              frame False {
              }
            }
          }
          frame "Maximize", "Maximized" {
            w303 = T1."Maximized" ("State")
            n146 = property class="VI"(reference=w309, error in=w308) -> (reference out=w306:refnum<vi>, error out=w307:errorcluster, "FP.State"=w305:T1)
            n147 = Not Equal?(x=w305, y=w303) -> (x != y?=w304:bool)
            n148 = case shown="True" w304 {
              tunnel: [w314 w315] -> w310
              tunnel: w307 -> [w313 w315]
              tunnel: w306 -> [w312 _]
              tunnel: w303 -> [w311 _]
              frame True {
                n149 = invoke class="VI" method="FP.Open"(reference=w312, error in=w313, "State"=w311) -> (error out=w314:errorcluster)  [unwired: 2 in, 4 out]
              }
              frame False {
              }
            }
          }
        }
        n150 = call <vilib>:"Add State(s) to Queue__JKI_lib_State_Machine.vi"("State(s) in (\"\")"=w250) -> ("States Out"=w249:string)  [unwired: 14 in]
      }
      frame "---------- Macro ----------" {
        # "Do not put any code in this frame.\n(It is a separator no-op. You can make a copy of this frame to create a new Macro frame)"
        n151 = call <vilib>:"Add State(s) to Queue__JKI_lib_State_Machine.vi"("State(s) in (\"\")"=w319) -> ("States Out"=w318:string)  [unwired: 14 in]
      }
      frame "Macro: Initialize" {
        # "Initialization Macro\n(This is called once, when the VI starts)"
        n152 = call <vilib>:"Add State(s) to Queue__JKI_lib_State_Machine.vi"("State(s) in Front (\"\")"="Data: Initialize\nInitialize Core Data\nEvents: Register\nUI: Initialize\nUI: Front Panel State >> Open", "State(s) in (\"\")"=w324) -> ("States Out"=w323:string)  [unwired: 13 in]
      }
      frame "Macro: Exit" {
        # "Exit Macro\n(This is called once, when the VI exits)"
        n153 = Unbundle By Name(w331) -> ("Core.Close Panel on Exit?"=w330:bool)
        n154 = Select(t="UI: Front Panel State >> Close", s=w330, f="") -> (s? t:f=w327:string)
        n155 = call <vilib>:"Add State(s) to Queue__JKI_lib_State_Machine.vi"("State(s) in (\"\")"=w327, "State(s) at Back (\"\")"="Data: Cleanup\nEvents: Unregister\nExit") -> ("States Out"=w325:string)  [unwired: 13 in]
        n156 = call <vilib>:"Add State(s) to Queue__JKI_lib_State_Machine.vi"("State(s) in Front (\"\")"=w325, "State(s) in (\"\")"=w334) -> ("States Out"=w333:string)  [unwired: 13 in]
      }
      frame "---------- DATABSE ----------" {
        # "Template Separator\n(You can make a copy of, or modify, this frame)"
        n157 = call <vilib>:"Add State(s) to Queue__JKI_lib_State_Machine.vi"("State(s) in (\"\")"=w338) -> ("States Out"=w337:string)  [unwired: 14 in]
      }
      frame "DATABASE: SAVE DATABASE" {
        # "Your code here.\n(You can make a copy of, or modify, this frame)"
        n158 = Unbundle By Name(w346) -> ("BATTERY EMULATOR"=w339:T4, "File paths.Model File path"=w342:path)
        n159 = Build Path(base path=w342, name or relative path="Battery Emulator.txt") -> (appended path=w343:path)
        n160 = Write to Binary File(file (use dialog)=w343, data=w339, error in=w345) -> (error out=w340:errorcluster)  [unwired: 3 in, 2 out]
        n161 = flat-sequence {
          tunnel: [w350] -> w341
          tunnel: w340 -> [w350]
          frame #0 {
            n162 = One Button Dialog(message="Battery Emulator data is Saved") -> ()  [unwired: 1 in, 1 out]
          }
        }
        n163 = call <vilib>:"Add State(s) to Queue__JKI_lib_State_Machine.vi"("State(s) in (\"\")"=w348) -> ("States Out"=w347:string)  [unwired: 14 in]
      }
      frame "DATABASE: READ DATABASE" {
        # "Your code here.\n(You can make a copy of, or modify, this frame)"
        n164 = Unbundle By Name(w371) -> ("BATTERY EMULATOR"=w365:T4, "File paths.Model File path"=w367:path)
        n165 = Build Path(base path=w367, name or relative path="Battery Emulator.txt") -> (appended path=w368:path)
        n166 = Read from Binary File(5:w365, 8:w370, 11:w368) -> (0:w366:errorcluster, 2:w364:T4)  [unwired: 3 in, 2 out]
        n167 = Cluster To Array(cluster=w364) -> (array=w363:string[])
        n168 = Index Array(array=w363) -> (element #1=w362:string, element #2=w361:string, element #3=w360:string, element #4=w359:string, element #5=w358:string, element #6=w357:string, element #7=w356:string, element #8=w355:string, element #9=w354:string, element #10=w353:string, element #11=w352:string)  [unwired: 11 in]
        n169 = property on="HVHC SELECTION" class="CmbBox"("Value"=w362) -> ()  [unwired: 2 in, 2 out]
        n170 = property on="CONTROL SELECTION" class="CmbBox"("Value"=w361) -> ()  [unwired: 2 in, 2 out]
        n171 = property on="CV VOLTAGE" class="Str"("Value"=w360) -> ()  [unwired: 2 in, 2 out]
        n172 = property on="CV CURRENT" class="Str"("Value"=w359) -> ()  [unwired: 2 in, 2 out]
        n173 = property on="CV POWER" class="Str"("Value"=w358) -> ()  [unwired: 2 in, 2 out]
        n174 = property on="CI VOLTAGE" class="Str"("Value"=w357) -> ()  [unwired: 2 in, 2 out]
        n175 = property on="CI CURRENT" class="Str"("Value"=w356) -> ()  [unwired: 2 in, 2 out]
        n176 = property on="CI POWER" class="Str"("Value"=w355) -> ()  [unwired: 2 in, 2 out]
        n177 = property on="CP CURRENT" class="Str"("Value"=w353) -> ()  [unwired: 2 in, 2 out]
        n178 = property on="CP VOLTAGE" class="Str"("Value"=w354) -> ()  [unwired: 2 in, 2 out]
        n179 = property on="CP POWER" class="Str"("Value"=w352) -> ()  [unwired: 2 in, 2 out]
        n180 = call <vilib>:"Add State(s) to Queue__JKI_lib_State_Machine.vi"("State(s) in (\"\")"=w373, "State(s) at Back (\"\")"="DATABASE: READ BATTERY DATA" ("State(s) at Back (\"\")")) -> ("States Out"=w372:string)  [unwired: 13 in]
      }
      frame "DATABASE: READ BATTERY DATA" {
        # "Your code here.\n(You can make a copy of, or modify, this frame)"
        n181 = call-poly <vilib>:"XNET Create Session.vi"("signal list"=refnum<k21>[] ["OutputCurrent\nFEV_150KW-R0", "OutputPower\nFEV_150KW-R0", "OutputVoltage\nFEV_150KW-R0", "ErrorControlSelErr\nFEV_150KW-R0", "ErrorNotInRemoteMode\nFEV_150KW-R0", "ErrorPowerSetOutofRange\nFEV_150KW-R0", "ErrorVoltSetOutofRange\nFEV_150KW-R0", "ErrorWrongHVSel\nFEV_150KW-R0", "PowerSwitchONStatus\nFEV_150KW-R0", "StatusDcpsFault\nFEV_150KW-R0", "StatusHCHV_selection\nFEV_150KW-R0", "HandShakeAcknowledge\nFEV_150KW-R0", "RemoteDisplaySelAck\nFEV_150KW-R0", "Select_CVCICPAck\nFEV_150KW-R0", "Select_HVHC_Ack\nFEV_150KW-R0", "CV_SetCurrentLimitAck\nFEV_150KW-R0", "CV_SetPowerLimitAck\nFEV_150KW-R0", "CV_SetVoltageAck\nFEV_150KW-R0", "UpdateCmdAcknowledge\nFEV_150KW-R0"] ("Sigs 2"), "interface"=refnum<k21> "CAN2" ("Select Interface"), "error in (no error)"=w397) -> ("session out"=w402:refnum<k21>, "error out"=w403:errorcluster)  [unwired: 1 in, 10 out]
        n182 = call <vilib>:"XNET Start.vi"("session in"=w402, "error in (no error)"=w403) -> ("session out"=w404:refnum<k21>, "error out"=w405:errorcluster)  [unwired: 12 in]
        n183 = call "Stall Data Flow.vim"("value in"=w405, "milliseconds to wait"=u32 1000) -> ("value out"=w401:errorcluster)  [unwired: 1 out]
        n184 = call-poly <vilib>:"XNET Read.vi"("session in"=w404, "error in (no error)"=w401) -> ("session out"=w377:refnum<k21>, "data"=w396:dbl[], "error out"=w378:errorcluster)  [unwired: 11 in]
        n185 = Number To Fractional String(number=w396) -> (F-format string=w393:string[])  [unwired: 3 in]
        n186 = Index Array(array=w393, index #1=13 ("index"), index #2=10 ("index")) -> (element #1=w394:string, element #2=w387:string)  [unwired: 1 in, 1 out]
        n187 = Index Array(array=w393) -> (element #1=w392:string, element #2=w391:string, element #3=w390:string)  [unwired: 3 in]
        n188 = call <vilib>:"XNET Stop.vi"("session in"=w377, "error in (no error)"=w378) -> ("session out"=w376:refnum<k21>, "error out"=w375:errorcluster)  [unwired: 12 in]
        n189 = Equal?(x=w387, y="224") -> (x = y?=w385:bool)
        n190 = case shown="\"228\"" w394 {
          tunnel: w392 -> [w415 w422 w429]
          tunnel: w391 -> [w414 w421 w428]
          tunnel: w390 -> [w413 w420 w427]
          tunnel: ["CV" "CI" "CP"] -> w388
          tunnel: [TRUE FALSE FALSE] -> w381
          tunnel: [FALSE FALSE TRUE] -> w380
          tunnel: [FALSE TRUE FALSE] -> w379
          frame "226", Default {
            "CV POWER" <- w413
            "CV VOLTAGE" <- w415
            "CV CURRENT" <- w414
          }
          frame "227" {
            "CI VOLTAGE" <- w422
            "CI CURRENT" <- w421
            "CI POWER" <- w420
          }
          frame "228" {
            "CP POWER" <- w427
            "CP CURRENT" <- w428
            "CP VOLTAGE" <- w429
          }
        }
        "CONTROL SELECTION" <- w388
        n191 = call <vilib>:"XNET Clear.vi"("session in"=w376, "error in (no error)"=w375) -> ("error out"=w374:errorcluster)  [unwired: 13 in]
        n192 = Select(t="HIGH CURRENT", s=w385, f="HIGH VOLTAGE") -> (s? t:f=→"HVHC SELECTION":string)
        n193 = property on="CI VOLTAGE" class="Str"("Visible"=w379) -> ()  [unwired: 2 in, 2 out]
        n194 = property on="CP VOLTAGE" class="Str"("Visible"=w380) -> ()  [unwired: 2 in, 2 out]
        n195 = property on="CP POWER" class="Str"("Visible"=w380) -> ()  [unwired: 2 in, 2 out]
        n196 = property on="CI CURRENT" class="Str"("Visible"=w379) -> ()  [unwired: 2 in, 2 out]
        n197 = property on="CP CURRENT" class="Str"("Visible"=w380) -> ()  [unwired: 2 in, 2 out]
        n198 = property on="CI POWER" class="Str"("Visible"=w379) -> ()  [unwired: 2 in, 2 out]
        n199 = call <vilib>:"Add State(s) to Queue__JKI_lib_State_Machine.vi"("State(s) in (\"\")"=w408) -> ("States Out"=w407:string)  [unwired: 14 in]
        n200 = property on="CV VOLTAGE" class="Str"("Visible"=w381) -> ()  [unwired: 2 in, 2 out]
        n201 = property on="CV CURRENT" class="Str"("Visible"=w381) -> ()  [unwired: 2 in, 2 out]
        n202 = property on="CV POWER" class="Str"("Visible"=w381) -> ()  [unwired: 2 in, 2 out]
      }
    }
  }
